vi "CameraSetParams.vi"(8 "error in (no error)":errorcluster, 10 "settings":T2={"exposure"=0.0, "external"=FALSE, "roi"={"left"=0, "top"=0, "right"=0, "bottom"=0}, "frames"=0, "binning"={"x"=1, "y"=1}}, 11 "CameraBase in":refnum<class "CameraBase.lvclass">) -> (0 "error out":errorcluster, 1 "roi_out":T1, 2 "attributes":variant[](array[variant]), 3 "CameraBase out":refnum<class "CameraBase.lvclass">)   [LabVIEW 2010, in "CameraBase.lvclass"]
uses:
  <userlib>/bias/classes/CameraBase/CameraBase.lvclass
  <userlib>/bias/subvis/ExposureSettings.ctl
  <userlib>/bias/subvis/ROI_rect.ctl
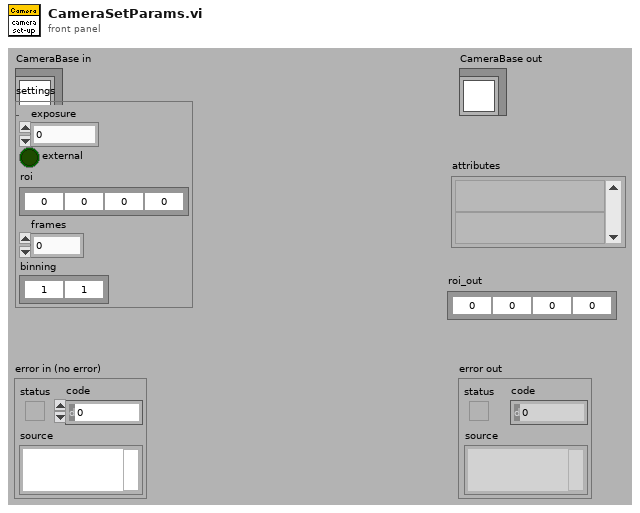
[diagram p1: front panel]
types:
  T1 = typedef "ROI_rect.ctl" = cluster{"left":i32, "top":i32, "right":i32, "bottom":i32}
  T2 = typedef "ExposureSettings.ctl" = cluster{"exposure":dbl, "external":bool, "roi":T1, "frames":i32, "binning":cluster{"x":u8, "y":u8}}
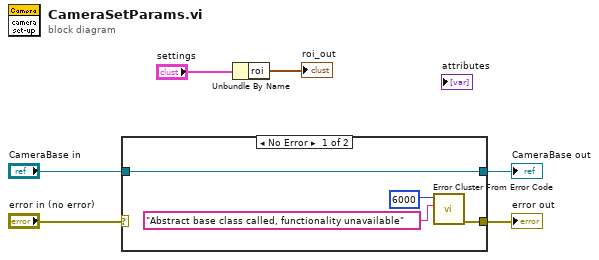
[diagram p0: block diagram]
diagram:
  n1 = case shown="No Error" "error in (no error)" {
    selector: "error in (no error)" -> [_ w12]
    tunnel: [w8 w12] -> w5
    tunnel: [w10 w11] -> w3
    tunnel: "CameraBase in" -> [w10 w11]
    frame No Error {
      n2 = call <vilib>:"Error Cluster From Error Code.vi"("error message (\"\")"="Abstract base class called, functionality unavailable" ("format string"), "error code (0)"=6000) -> ("error out"=w8:errorcluster)  [unwired: 7 in]
    }
    frame Error {
    }
  }
  "error out" <- w5
  "CameraBase out" <- w3
  n3 = Unbundle By Name("settings") -> ("roi"=→"roi_out":T1)
